vi "Delete Project Temporary Files.vi"(8 "error in (no error)":errorcluster, 11 "Project Path":path) -> (0 "error out":errorcluster)   [LabVIEW 2021, in "Build Script Common.lvlib"]
uses:
  Build Script Common.lvlib
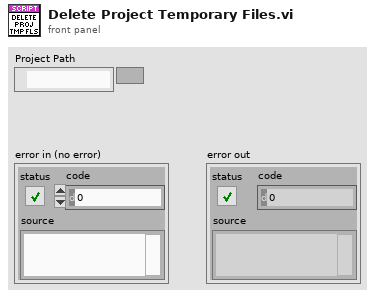
[diagram p1: front panel]
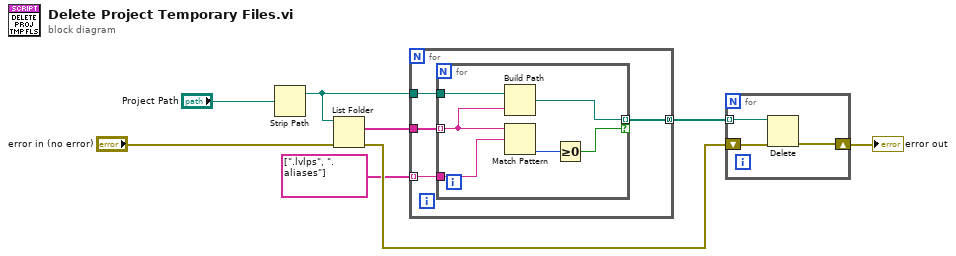
[diagram p0: block diagram]
diagram:
  n1 = Strip Path(path="Project Path") -> (stripped path=w3:path)  [unwired: 1 out]
  n2 = List Folder(path=w3, error in="error in (no error)") -> (filenames=w1:string[], error out=w5:errorcluster)  [unwired: 2 in, 2 out]
  n3 = for {
    tunnel: w1 -> [w12]
    tunnel: string[] [".lvlps", ".aliases"] -> [w11] mode=indexing
    tunnel: [w10] -> w4 mode=concatenating
    tunnel: w3 -> [w9]
    n4 = for {
      tunnel: [w13] -> w10 mode=indexing if=w18
      tunnel: w11 -> [w17]
      tunnel: w12 -> [w15] mode=indexing
      tunnel: w9 -> [w14]
      n5 = Build Path(base path=w14, name or relative path=w15) -> (appended path=w13:path)
      n6 = Match Pattern(string=w15, regular expression=w17) -> (offset past match=w16:i32)  [unwired: 1 in, 3 out]
      n7 = Greater Or Equal To 0?(x=w16) -> (x >= 0?=w18:bool)
    }
  }
  n8 = for {
    tunnel: w4 -> [w21] mode=indexing
    shift-right: [w19] -> w8
    shift-left: w5 -> [w20]
    n9 = Delete(path (use dialog)=w21, error in=w20) -> (error out=w19:errorcluster)  [unwired: 3 in, 2 out]
  }
  "error out" <- w8
